vi "set_config_cluster.vi"(8 "error in (no error)":errorcluster, 10 "config cluster variant":variant, 11 "TraceProcessorDL090628DSS in":refnum<class "TraceProcessorDL090628DSS.lvclass">) -> (0 "error out":errorcluster, 3 "TraceProcessorDL090628DSS out":refnum<class "TraceProcessorDL090628DSS.lvclass">)   [LabVIEW 2010, in "TraceProcessorDL090628DSS.lvclass"]
uses:
  TraceProcessorDL090628DSS.lvclass
  TraceProcessorDL090628DSS.lvclass/TraceProcessorDL090628DSS.ctl
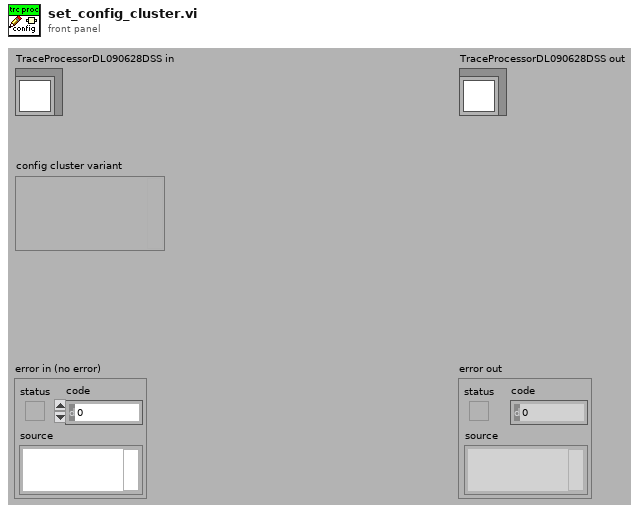
[diagram p1: front panel]
types:
  T1 = typedef "TraceProcessorDL090628DSS.lvclass/config_data_cluster.ctl" = cluster{"baseline sampling pixels":i32}
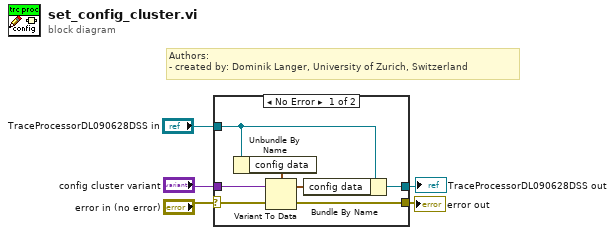
[diagram p0: block diagram]
diagram:
  # "Authors: \n- created by: Dominik Langer, University of Zurich, Switzerland"
  n1 = case shown="No Error" "error in (no error)" {
    selector: "error in (no error)" -> [w10 w13]
    tunnel: "TraceProcessorDL090628DSS in" -> [w8 w14]
    tunnel: [w7 w13] -> w1
    tunnel: [w6 w14] -> w2
    tunnel: "config cluster variant" -> [w9 _]
    frame No Error {
      n2 = Unbundle By Name(w8) -> ("config data"=w12:T1)
      n3 = Variant To Data(error in=w10, Variant=w9, type=w12) -> (error out=w7:errorcluster, data=w11:T1)
      n4 = Bundle By Name(cluster=w8, "config data"=w11) -> (w6:refnum<class "TraceProcessorDL090628DSS.lvclass">)
    }
    frame Error {
    }
  }
  "error out" <- w1
  "TraceProcessorDL090628DSS out" <- w2
